vi "Read OD data backup.vi"(4 "OD num":dbl) -> (1 "OD data":dbl[][](array[numeric]) caption="所有行" format="%0.3f")   [LabVIEW 2013]
uses:
  <vilib>/Utility/file.llb/Read From Spreadsheet File (DBL).vi
panel:
  out "路径":path
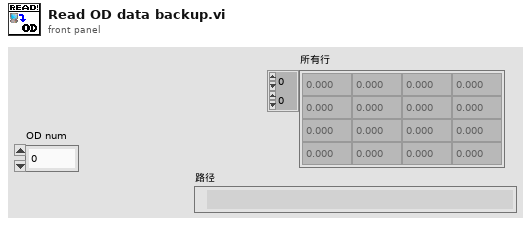
[diagram p1: front panel]
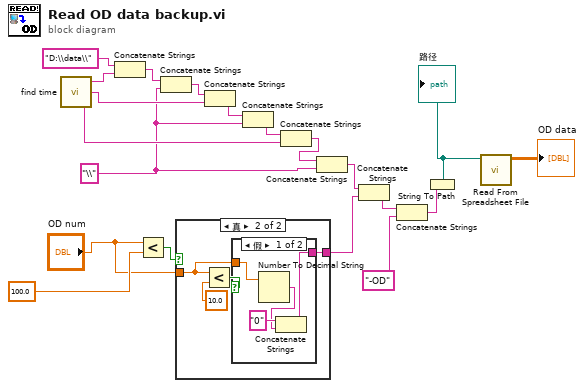
[diagram p0: block diagram]
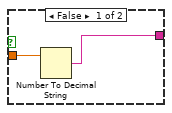
[diagram p2: hidden frame]
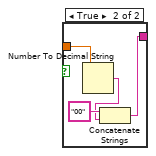
[diagram p3: hidden frame]
diagram:
  w11 = "\\" ("字符串")
  n1 = call "find time.vi"() -> ("day"=w13:string, "month"=w16:string, "year"=w19:string)  [unwired: 3 in]
  n2 = Concatenate Strings("D:\\data\\", w19) -> (w18:string)
  n3 = Less?(x="OD num", y=100.0) -> (x < y?=w3:bool)
  n4 = Concatenate Strings(w18, w11) -> (w17:string)
  n5 = case shown="真" w3 {
    tunnel: "OD num" -> [w22 w24]
    tunnel: [w21 w23] -> w1
    frame False {
      n6 = Number To Decimal String(number=w22) -> (decimal integer string=w21:string)  [unwired: 1 in]
    }
    frame True {
      n7 = Less?(x=w24, y=10.0) -> (x < y?=w25:bool)
      n8 = case shown="假" w25 {
        tunnel: w24 -> [w29 w34]
        tunnel: [w27 w31] -> w23
        frame False {
          n9 = Number To Decimal String(number=w29) -> (decimal integer string=w28:string)  [unwired: 1 in]
          n10 = Concatenate Strings("0" ("字符串"), w28) -> (w27:string)
        }
        frame True {
          n11 = Number To Decimal String(number=w34) -> (decimal integer string=w32:string)  [unwired: 1 in]
          n12 = Concatenate Strings("00" ("字符串"), w32) -> (w31:string)
        }
      }
    }
  }
  n13 = Concatenate Strings(w17, w16) -> (w15:string)
  n14 = Concatenate Strings(w15, w11) -> (w14:string)
  n15 = Concatenate Strings(w14, w13) -> (w12:string)
  n16 = Concatenate Strings(w12, w11) -> (w10:string)
  n17 = Concatenate Strings(w10, w1) -> (w7:string)
  n18 = Concatenate Strings(w7, "-OD" ("字符串")) -> (w5:string)
  n19 = String To Path(string=w5) -> (path=w9:path)
  "路径" <- w9
  n20 = call-poly <vilib>:"Read From Spreadsheet File.vi"("file path (dialog if empty)"=w9) -> ("all rows"=→"OD data":dbl[][])  [unwired: 6 in, 4 out]
